vi "Sub_MotorC.vi"(1 "C":i32) -> (0 "문자열":string)   [LabVIEW 2013]
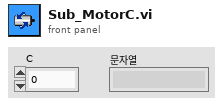
[diagram p1: front panel]
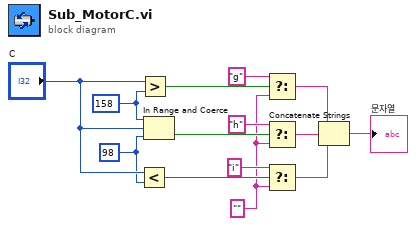
[diagram p0: block diagram]
diagram:
  w1 = ""
  w10 = 98
  w9 = 158
  n1 = Less?(x="C", y=w10) -> (x < y?=w11:bool)
  n2 = Greater?(x="C", y=w9) -> (0:w13:bool)
  n3 = In Range and Coerce(upper limit=w9, x="C", lower limit=w10) -> (In Range?=w12:bool)  [unwired: 1 out]
  n4 = Select(t="g", s=w13, f=w1) -> (s? t:f=w5:string)
  n5 = Select(t="h", s=w12, f=w1) -> (s? t:f=w4:string)
  n6 = Select(t="i", s=w11, f=w1) -> (s? t:f=w3:string)
  n7 = Concatenate Strings(w5, w4, w3) -> (→"문자열":string)
